vi "InstrumentReferences.vi"() -> ()   [LabVIEW 2019]
panel:
  in  "ESP300 COM Port":refnum<visa-resource-name>="COM4" caption="COM Port"
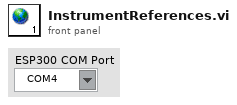
[diagram p1: front panel]
diagram:
